vi "CAN SignalsSorted By StartBit.vi"(8 "Fehler (Eingang, kein Fehler)":errorcluster, 11 "selected SAE J-1939 Signals":refnum<k21>[](array[refnum])) -> (0 "Fehler (Ausgang)":errorcluster, 3 "sorted selected SAE J-1939 Signals":refnum<k21>[](array[refnum]))   [LabVIEW 2020, in "CAN Konfig.lvlib"]
uses:
  CAN Konfig.lvlib
  2761aa41-52dd-488d-8ddd-b184672d60a4.vi
  <vilib>/Array/Sort 2D Array - Pop Stack.vi
  <vilib>/Array/Sort 2D Array - Push Stack.vi
  <resource>/objmgr/xnet.rc
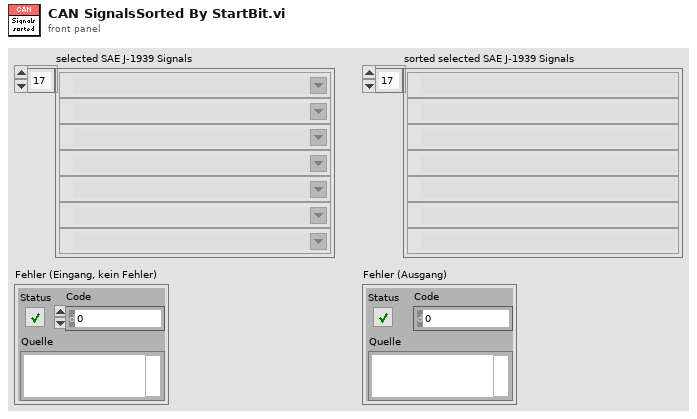
[diagram p1: front panel]
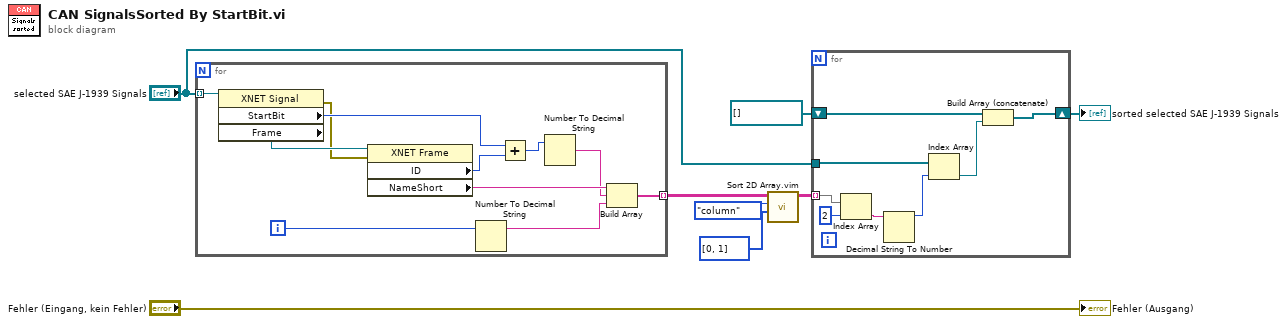
[diagram p0: block diagram]
diagram:
  n1 = for {
    tunnel: "selected SAE J-1939 Signals" -> [w19] mode=indexing
    tunnel: [w14] -> w4 mode=indexing
    i -> [w15]
    n2 = property class="XNET Signal"(reference=w19) -> (error out=w13:errorcluster, "StartBit"=w17:u32, "Frame"=w18:refnum<k21>)  [unwired: 1 in, 1 out]
    n3 = property class="XNET Frame"(reference=w18, error in=w13) -> ("ID"=w16:u32, "NameShort"=w12:string)  [unwired: 2 out]
    n4 = Number To Decimal String(number=w15) -> (decimal integer string=w11:string)  [unwired: 1 in]
    n5 = Add(x=w17, y=w16) -> (x+y=w9:u32)
    n6 = Number To Decimal String(number=w9) -> (decimal integer string=w10:string)  [unwired: 1 in]
    n7 = Build Array(w12, w10, w11) -> (w14:string[])
  }
  n8 = call "Sort 2D Array.vim"("index"=i32[] [0, 1], "dimension to index (column)"=enum16{"column", "row"}."column", "2D array"=w4) -> ("sorted 2D array"=w1:string[][])  [unwired: 7 in, 1 out]
  n9 = for {
    tunnel: w1 -> [w27] mode=indexing
    tunnel: "selected SAE J-1939 Signals" -> [w25]
    shift-right: [w22] -> w6
    shift-left: refnum<k21>[] [] -> [w21]
    n10 = Index Array(array=w27, index=2 ("Index")) -> (element=w24:string)
    n11 = Decimal String To Number(string=w24) -> (number=w20:i32)  [unwired: 2 in, 1 out]
    n12 = Index Array(array=w25, index=w20) -> (element=w23:refnum<k21>)
    n13 = Build Array (concatenate)(w21, w23) -> (w22:refnum<k21>[])
  }
  "sorted selected SAE J-1939 Signals" <- w6
  "Fehler (Ausgang)" <- "Fehler (Eingang, kein Fehler)"
